vi "onCreateListener.vi"(6 "timeout (ms)":i32=100, 8 "error in (no error)":errorcluster, 10 "Configuration":refnum<class "LocalQueueConnection.lvclass">) -> (0 "error out":errorcluster, 3 "Listener":refnum<class "Connection.lvclass">)   [LabVIEW 2013, in "MQTT_Queue.lvlib" / "LocalQueueConnection.lvclass"]
uses:
  LocalQueueConnection.lvclass
  MQTT_Connection/Connection/Connection.lvclass
  LocalQueueConnection.lvclass/LocalQueueConnection.ctl
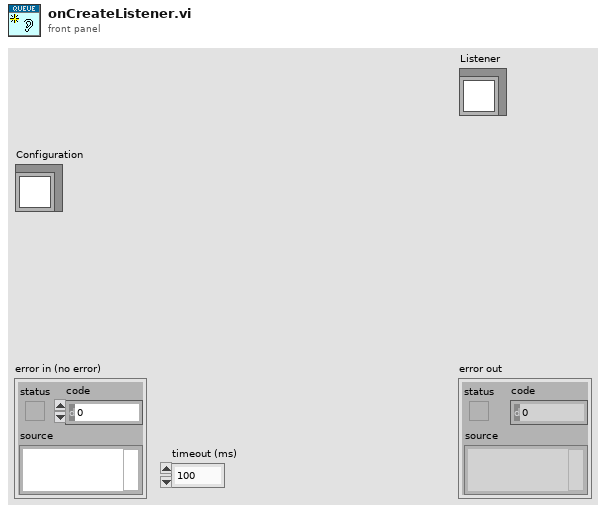
[diagram p1: front panel]
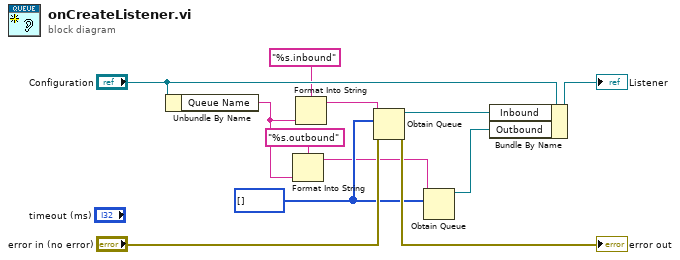
[diagram p0: block diagram]
diagram:
  w7 = u8[] [] ("Bytes Stream")
  n1 = Unbundle By Name("Configuration") -> ("Queue Name"=w3:string)
  n2 = Format Into String(format string="%s.outbound", w3) -> (resulting string=w1:string)  [unwired: 2 in, 1 out]
  n3 = Format Into String(format string="%s.inbound", w3) -> (resulting string=w5:string)  [unwired: 2 in, 1 out]
  n4 = Obtain Queue(name (unnamed)=w5, element data type=w7, error in (no error)="error in (no error)") -> (queue out=w11:refnum<queue>, error out=→"error out":errorcluster)  [unwired: 2 in, 1 out]
  n5 = Obtain Queue(name (unnamed)=w1, element data type=w7) -> (queue out=w6:refnum<queue>)  [unwired: 3 in, 2 out]
  n6 = Bundle By Name(cluster="Configuration", "Inbound"=w11, "Outbound"=w6) -> (→"Listener":refnum<class "LocalQueueConnection.lvclass">)
